vi "Enqueue (Single).vi"(6 "timeout in ms (-1)":i32=-1, 7 "Priority Message? Array":bool, 8 "error in (no error)":errorcluster, 9 "Message Data Array":variant, 10 "States":T1=enum."Default", 11 "Message Queue":refnum<queue>) -> (0 "error out":errorcluster, 3 "dup Message Queue":refnum<queue>)   [LabVIEW 2019, in "Status.lvlib"]
doc: "For a regular message, enqueue the message. For a priority message, enqueue it at the front of the queue."
uses:
  Status.lvlib
  Queue Type.ctl
  State Name.ctl
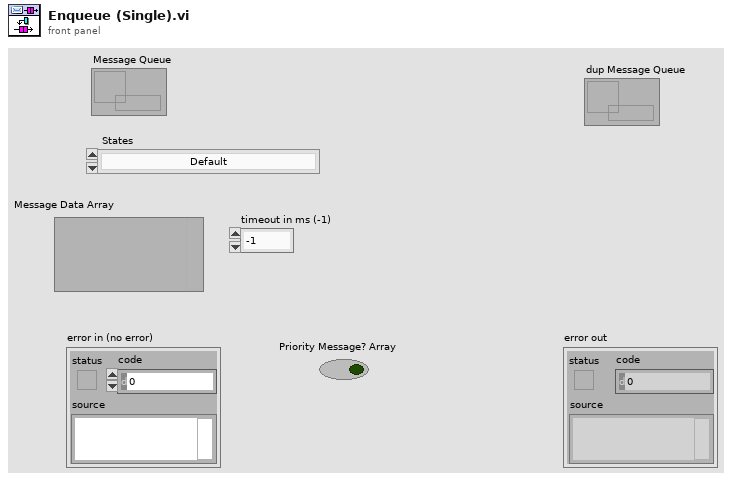
[diagram p1: front panel]
types:
  T1 = typedef "Status.lvlib/State Name.ctl" = enum16{"Initialize", "Update Progress Bar", "Update Status Bar", "Set Cursor Busy", "Unset Cursor Busy", "Error", "Default", "Exit"}
  T2 = typedef "Status.lvlib/Queue Type.ctl" = cluster{"Custom State Name":string, "Defined State Name":T1, "Call Chain":string[], "Message Data":variant}
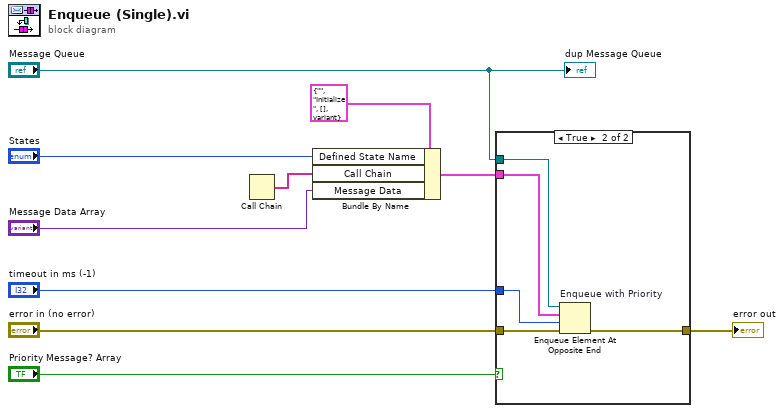
[diagram p0: block diagram]
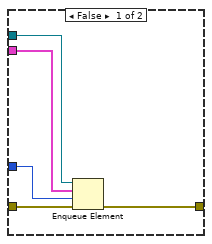
[diagram p2: hidden frame]
diagram:
  n1 = Call Chain() -> (call chain=w2:string[])
  n2 = Bundle By Name(cluster=T2 {"Custom State Name"="", "Defined State Name"=enum."Initialize", "Call Chain"=[], "Message Data"=variant} ("Message Cluster"), "Defined State Name"="States", "Call Chain"=w2, "Message Data"="Message Data Array") -> (w4:T2)
  n3 = case shown="True" "Priority Message? Array" {
    tunnel: "error in (no error)" -> [w15 w20]
    tunnel: [w14 w19] -> w8
    tunnel: "Message Queue" -> [w13 w18]
    tunnel: w4 -> [w12 w17]
    tunnel: "timeout in ms (-1)" -> [w11 w16]
    frame False {
      n4 = Enqueue Element(queue=w13, element=w12, timeout in ms (-1)=w11, error in (no error)=w15) -> (error out=w14:errorcluster)  [unwired: 2 out]
    }
    frame True {
      n5 = Enqueue Element At Opposite End "Enqueue with Priority"(queue=w18, element=w17, timeout in ms (-1)=w16, error in (no error)=w20) -> (error out=w19:errorcluster)  [unwired: 2 out]
    }
  }
  "error out" <- w8
  "dup Message Queue" <- "Message Queue"
